vi "get_notification_from_queue.vi"(0 "Error in":errorcluster, 1 "Queue in":refnum<queue>) -> (2 "Error out":errorcluster, 3 "Should act":bool, 4 "Queue out":refnum<queue>)   [LabVIEW 2015]
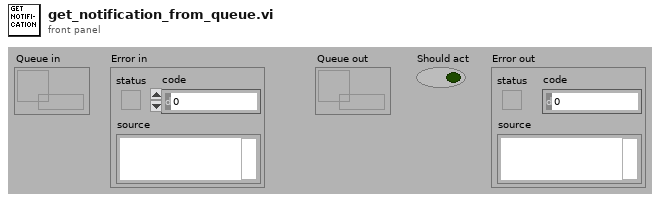
[diagram p1: front panel]
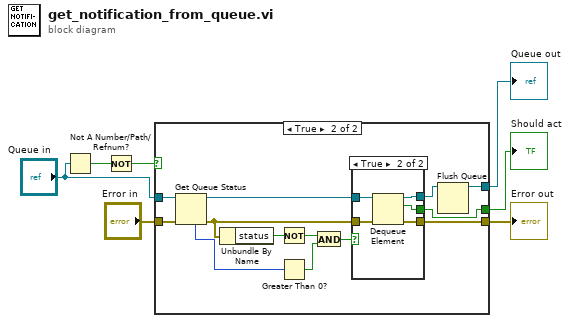
[diagram p0: block diagram]
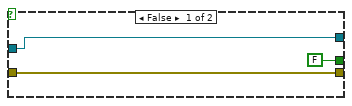
[diagram p2: hidden frame]
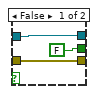
[diagram p3: hidden frame]
diagram:
  n1 = Not A Number/Path/Refnum?(number/path/refnum="Queue in") -> (NaN/Path/Refnum?=w2:bool)
  n2 = Not(x=w2) -> (.not. x?=w1:bool)
  n3 = case shown="True" w1 {
    tunnel: "Error in" -> [w9 w23]
    tunnel: [w9 w22] -> w6
    tunnel: [FALSE w21] -> w5
    tunnel: "Queue in" -> [w10 w14]
    tunnel: [w10 w12] -> w4
    frame False {
    }
    frame True {
      n4 = Get Queue Status(queue=w14, error in (no error)=w23) -> (queue out=w19:refnum<queue>, error out=w11:errorcluster, # elements in queue=w15:i32)  [unwired: 1 in, 5 out]
      n5 = Unbundle By Name(w11) -> ("status"=w16:bool)
      n6 = Not(x=w16) -> (.not. x?=w17:bool)
      n7 = Greater Than 0?(x=w15) -> (x > 0?=w18:bool)
      n8 = And(x=w17, y=w18) -> (x .and. y?=w20:bool)
      n9 = case shown="True" w20 {
        tunnel: w19 -> [w26 w31]
        tunnel: [w26 w30] -> w13
        tunnel: [FALSE w29] -> w21
        tunnel: [w24 w28] -> w22
        tunnel: w11 -> [w24 w27]
        frame False {
        }
        frame True {
          n10 = Dequeue Element(queue=w31, error in (no error)=w27) -> (queue out=w30:refnum<queue>, element=w29:bool, error out=w28:errorcluster)  [unwired: 1 in, 1 out]
        }
      }
      n11 = Flush Queue(queue=w13) -> (queue out=w12:refnum<queue>)  [unwired: 1 in, 2 out]
    }
  }
  "Error out" <- w6
  "Should act" <- w5
  "Queue out" <- w4
